vi "qSMR.vi"(0 "System no.":i32=1 min=1 max=4 step=1, 2 "Axes to query":string[](array[string]), 5 "error in":errorcluster) -> (14 "Remaining steps":dbl[](array[numeric]) format="%.6f", 19 "error out":errorcluster)   [LabVIEW 2020]
doc: "SMR? (Get Remaining Steps)\n\nDescription\nQueries the current number and direction of the steps still to be moved for the axes.\n\nFormat\nSMR?[ <AxisID>]\n\nArguments\nSMR? without arguments queries all axes of the controller.\n<AxisID>\nAn axis of the controller\nThe available axes can be queried with USG? SYS. The axes for which the command is permitted \ncan be queried with USG? CMD SMR?.\nPossible values: Alias of the axis (p. 94) \n\nResponse\n{<AxisID>\"=\"<RemainingSteps> LF} \n<RemainingSteps>\nThe current number and direction of the steps still to be moved\nThe data format is float.\nThe sign indicates the direction of motion.\nPossible values: Dependent on the controller\n\nExample\nSee SMV\n\nNotes\nThe SMV command (p. 56) specifies the number and direction of the steps to be moved.\nThe SMV? command (p. 59) queries the number and direction of the commanded steps.\nComparison of the behavior of SMV? and SMR? when displaying the number of steps: \n1) Execution of the \ncommanded steps is in \nprogress.\n2) Execution of the \ncommanded steps is \ncomplete.\n3) While executing the \nsteps from the previous \ncommand, a new number \nof steps is commanded.\nSMV? The full number of \ncommanded steps is \ndisplayed and remains \nconstant.\nAfter executing the last \nstep, the display switches \nto zero.\nThe display of the steps \nswitches to the new \ncommanded value.\nThe behavior described in \n1) and 2) is repeated. SMR? The displayed number of \nsteps decreases stepwise \nas the steps are executed.\nAfter executing the last \nstep, the display ends at \nzero.\nSTP (p. 65) and HLT (p. 19) set the number of commanded steps to zero.\n\nUser command level\nUSR"
panel:
  # "SMR? (Get Remaining Steps)\n\nQueries the current number and direction of the steps still to be moved for the axes."
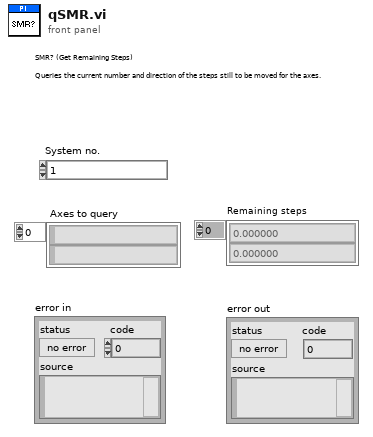
[diagram p1: front panel]
types:
  T1 = typedef "Syntax.ctl" = enum16{"GCS 1.0", "GCS 2.0", "GCS 3.0"}
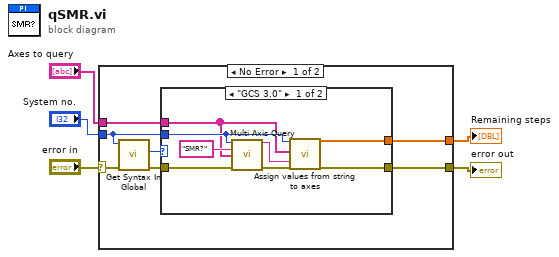
[diagram p0: block diagram]
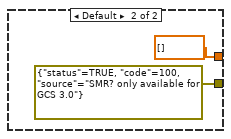
[diagram p2: hidden frame]
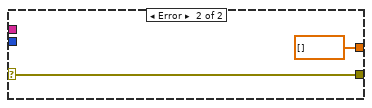
[diagram p3: hidden frame]
diagram:
  n1 = case shown="No Error" "error in" {
    selector: "error in" -> [w12 w24]
    tunnel: [w9 w24] -> w2
    tunnel: "System no." -> [w8 _]
    tunnel: [w7 dbl[] [] ("Target position")] -> w1
    tunnel: "Axes to query" -> [w6 _]
    frame No Error {
      n2 = call "Get Syntax In Global.vi"("error in"=w12, "System no."=w8) -> ("error out"=w10:errorcluster, "Syntax"=w11:T1)  [unwired: 8 in]
      n3 = case shown="\"GCS 3.0\"" w11 {
        tunnel: [w13 errorcluster {"status"=TRUE, "code"=100, "source"="SMR? only available for GCS 3.0"} ("error out")] -> w9
        tunnel: w10 -> [w17 _]
        tunnel: w6 -> [w15 _]
        tunnel: w8 -> [w16 _]
        tunnel: [w14 dbl[] [] ("Target position")] -> w7
        frame "GCS 3.0" {
          n4 = call "Multi Axis Query.vi"("System no."=w16, "Command"="SMR?", "Axis"=w15, "error in (no error)"=w17) -> ("Answer"=w19:string, "error out"=w20:errorcluster)  [unwired: 10 in]
          n5 = call "Assign values from string to axes.vi"("System no."=w16, "Queried axes"=w15, "Input String"=w19, "error in"=w20) -> ("Values"=w14:dbl[], "error out"=w13:errorcluster)  [unwired: 2 in, 12 out]
        }
        frame Default {
        }
      }
    }
    frame Error {
    }
  }
  "error out" <- w2
  "Remaining steps" <- w1
